vi "specu1a 1.0.0 Write PUnit Information.vi"(0 "Device Handle":i32, 2 "P Info in":T1={"UnitID"="", "Sensor Name"="", "Serial Number"="", "Reserved"="", "Wave Upper"=630, "Wave Lower"=1050}, 3 "error in (no error)":errorcluster, 4 "mark":i8 format="%.0x") -> (5 "Device Handle out":i32, 6 "P Info out":T1={"UnitID"="", "Sensor Name"="", "Serial Number"="", "Reserved"="", "Wave Upper"=630, "Wave Lower"=1050}, 7 "error out":errorcluster)   [LabVIEW 2010]
uses:
  Controls/specu1a 1.0.0 Product Information.ctl
  WINDOWS/SYSTEM32/DRIVERS/specu1a.dll
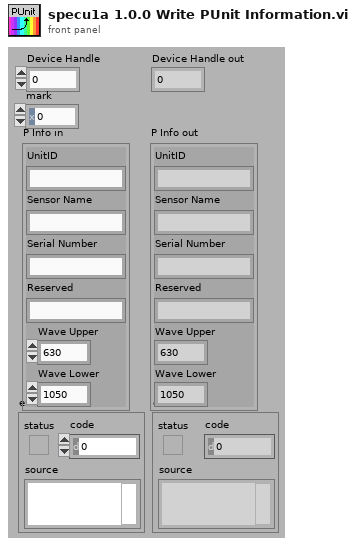
[diagram p1: front panel]
types:
  T1 = typedef "specu1a 1.0.0 Product Information.ctl" = cluster{"UnitID":string, "Sensor Name":string, "Serial Number":string, "Reserved":string, "Wave Upper":u16, "Wave Lower":u16}
  T2 = cluster{"UnitID":cluster{u8, u8, u8, u8, u8, u8, u8, u8}, "Sensor Name":cluster{u8, u8, u8, u8, u8, u8, u8, u8, u8, u8, u8, u8, u8, u8, u8, u8}, "Serial Number":cluster{u8, u8, u8, u8, u8, u8, u8, u8}, "Reserved":cluster{u8, u8, u8, u8, u8, u8, u8, u8}, "Wave Upper":u16, "Wave Lower":u16}
  T3 = typedef "specu1a 1.0.0 Error codes.ctl" = enum16{"INVALID_HANDLE_VALUE", "USBDEV_SUCCESS", "USBDEV_INVALID_HANDLE", "USBDEV_UNSUCCESS", "USBDEV_INVALID_VALUE", "USBDEV_CHECK_NORMAL", "USBDEV_CHECK_INVALID", "USBDEV_CHECK_REMOVE", "USBDEV_CHECK_OTHER", "USBDEV_RESET_ERROR", "USBDEV_BULKSIZE_ERROR", "USBDEV_BULK_READ_ERROR", "USBDEV_BULK_NOT_UPDATED", "USBDEV_TIME_OVER_ERROR", "USBDEV_TIME_UNDER_ERROR", "USBDEV_TIME_SET_ERROR", "USBDEV_SET_GAIN_ERROR", "USBDEV_GET_TEMP_ERROR", "USBDEV_SET_TRIGGER_ERROR", "USBDEV_RW_EEP_ADDR_ERROR", "USBDEV_RW_EEP_SIZE_ERROR", "USBDEV_RW_EEP_OVER_ERROR", "USBDEV_RW_EEP_ERROR", "UNITID_PRODUCTID_CONFLICT", "UNKNOWN_ERROR"}
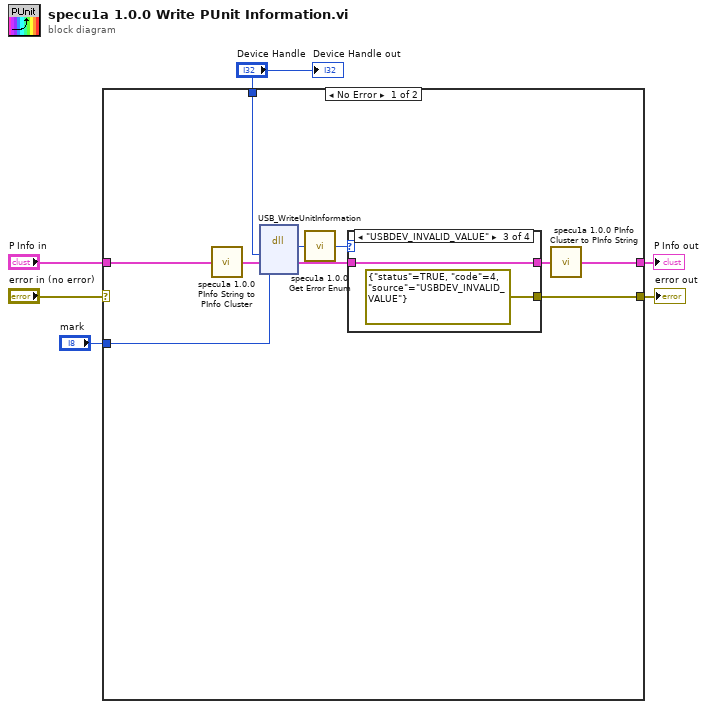
[diagram p0: block diagram]
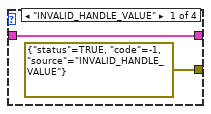
[diagram p2: hidden frame]
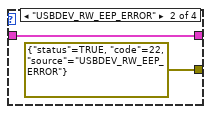
[diagram p3: hidden frame]
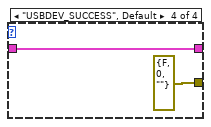
[diagram p4: hidden frame]
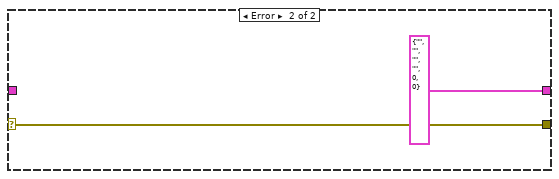
[diagram p5: hidden frame]
diagram:
  n1 = case shown="No Error" "error in (no error)" {
    selector: "error in (no error)" -> [_ w26]
    tunnel: [w15 w26] -> w5
    tunnel: [w13 T1 {"UnitID"="", "Sensor Name"="", "Serial Number"="", "Reserved"="", "Wave Upper"=0, "Wave Lower"=0} ("output cluster 2")] -> w1
    tunnel: "Device Handle" -> [w11 _]
    tunnel: "P Info in" -> [w12 _]
    tunnel: "mark" -> [w7 _]
    frame No Error {
      n2 = call "specu1a 1.0.0 PInfo String to PInfo Cluster.vi"("Unit Information in"=w12) -> ("output cluster"=w9:T2)
      n3 = dll-call lib="C:/WINDOWS/SYSTEM32/DRIVERS/specu1a.dll" fn="USB_WriteUnitInformation" label="1.0.0 Write unit information"("Device Handle"=w11, "output cluster"=w9, "mark"=w7) -> (w10:u16, "output cluster"=w8:T2)  [unwired: 5 in, 2 out]
      n4 = call "specu1a 1.0.0 Get Error Enum.vi"("Error Code in"=w10) -> ("Specu1a 1.0.0 Error code out"=w16:T3)  [unwired: 4 in]
      n5 = case shown="\"USBDEV_INVALID_VALUE\"" w16 {
        tunnel: [w17 w19 w21 w23] -> w14
        tunnel: [errorcluster {"status"=TRUE, "code"=-1, "source"="INVALID_HANDLE_VALUE"} ("error out") errorcluster {"status"=TRUE, "code"=22, "source"="USBDEV_RW_EEP_ERROR"} ("error out") errorcluster {"status"=TRUE, "code"=4, "source"="USBDEV_INVALID_VALUE"} ("error out") errorcluster {"status"=FALSE, "code"=0, "source"=""} ("error out")] -> w15
        tunnel: w8 -> [w17 w19 w21 w23]
        frame "INVALID_HANDLE_VALUE" {
        }
        frame "USBDEV_RW_EEP_ERROR" {
        }
        frame "USBDEV_INVALID_VALUE" {
        }
        frame "USBDEV_SUCCESS", Default {
        }
      }
      n6 = call "specu1a 1.0.0 PInfo Cluster to PInfo String.vi"("output cluster"=w14) -> ("output cluster 2"=w13:T1)
    }
    frame Error {
    }
  }
  "error out" <- w5
  "P Info out" <- w1
  "Device Handle out" <- "Device Handle"
